vi "test_Find Equation Variables_2 values tested.vi"(8 "error in (no error)":errorcluster, 11 "TestCase in":refnum<class "Instrument Addon Unit Tests.lvclass">) -> (0 "error out":errorcluster, 3 "TestCase out":refnum<class "Instrument Addon Unit Tests.lvclass">)   [LabVIEW 2018, in "Instrument Addon Unit Tests.lvclass"]
uses:
  Instrument Addon Unit Tests.lvclass
  <vilib>/addons/_JKI Toolkits/VI Tester/TestCase.llb/TestCase.lvclass
  Addon/Addon System Explorer/Instrument Addon System Explorer.lvlib
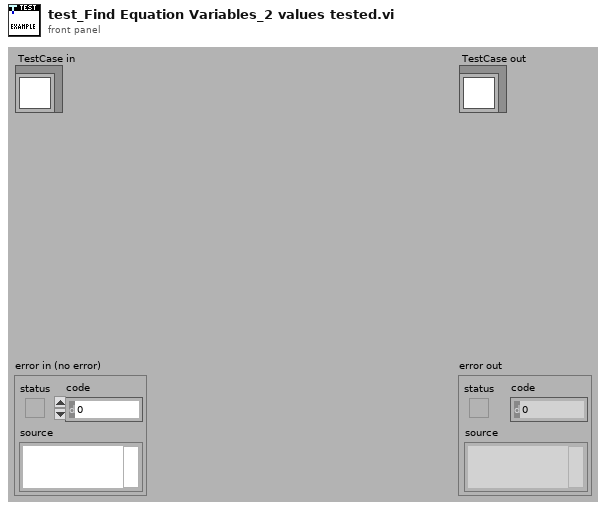
[diagram p1: front panel]
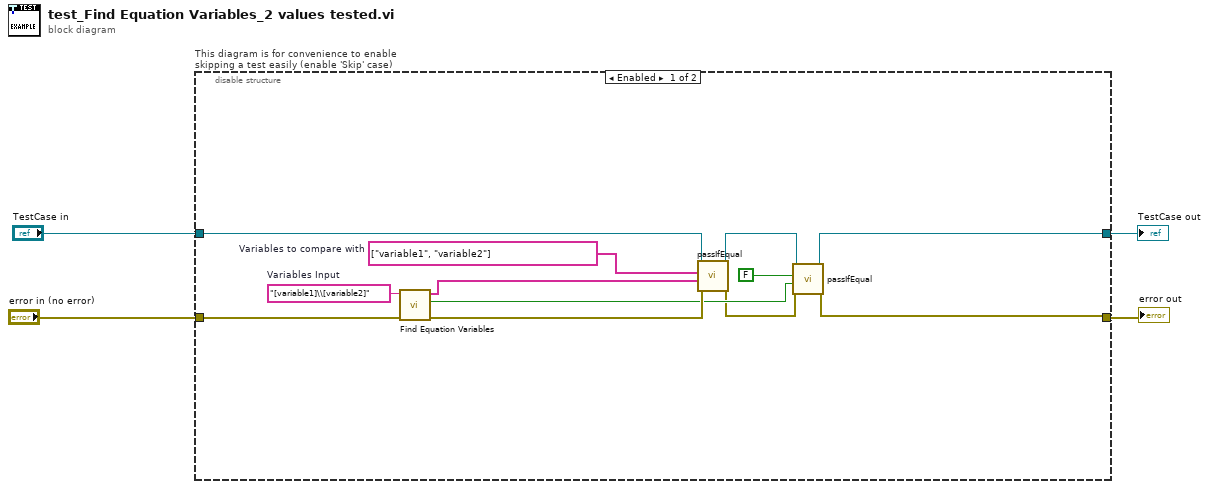
[diagram p0: block diagram]
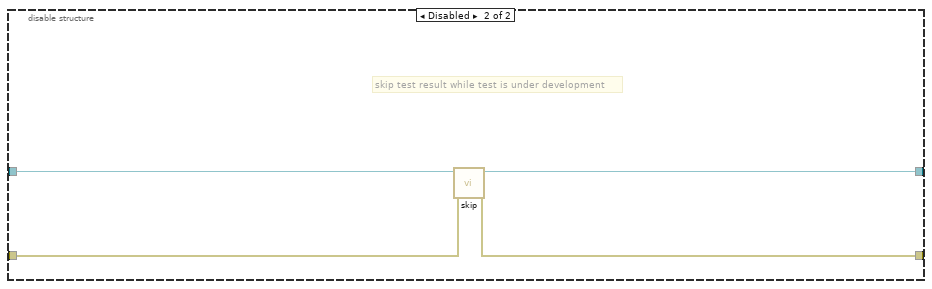
[diagram p2: hidden frame]
diagram:
  n1 = disable-structure "This diagram is for convenience to enable skipping a test easily (enable 'Skip' case)" shown="Enabled" {
    disable-tunnel: "TestCase in" -> [w11 w20]
    disable-tunnel: [w7 w18] -> w1
    disable-tunnel: [w5 w19] -> w3
    disable-tunnel: "error in (no error)" -> [w16 w17]
    frame Enabled {
      w12 = string[] ["variable1", "variable2"]  # Variables to compare with
      w13 = "[variable1]\\[variable2]"  # Variables Input
      n2 = call "Find Equation Variables.vi"("error in (no error)"=w16, "Command"=w13) -> ("error out"=w15:errorcluster, "Duplicate?"=w10:bool, "Variables"=w14:string[])  [unwired: 7 in]
      n3 = call-dynamic "passIfEqual.vi"("error in (no error)"=w15, "y"=w14, "x"=w12, "TestCase in"=w11) -> ("error out"=w6:errorcluster, "TestCase out"=w8:refnum<class "Instrument Addon Unit Tests.lvclass">)  [unwired: 6 in]
      n4 = call-dynamic "passIfEqual.vi"("error in (no error)"=w6, "y"=w10, "x"=FALSE, "TestCase in"=w8) -> ("error out"=w5:errorcluster, "TestCase out"=w7:refnum<class "Instrument Addon Unit Tests.lvclass">)  [unwired: 6 in]
    }
    frame Disabled {
      # "skip test result while test is under development"
      n5 = call <vilib>:"skip.vi"("error in (no error)"=w17, "TestCase in"=w20) -> ("error out"=w19:errorcluster, "TestCase out"=w18:refnum<class "Instrument Addon Unit Tests.lvclass">)  [unwired: 8 in]
    }
  }
  "error out" <- w3
  "TestCase out" <- w1
